vi "Count_looped.vi"(7 "Reset?":bool[](array[boolean]), 11 "Input array":dbl[](array[numeric])) -> (3 "Output array":dbl[](array[numeric]))   [LabVIEW 2018]
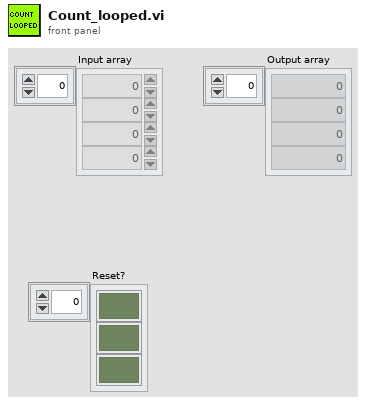
[diagram p1: front panel]
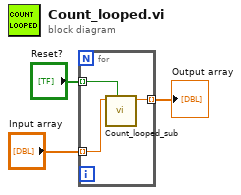
[diagram p0: block diagram]
diagram:
  n1 = for {
    tunnel: "Input array" -> [w5] mode=indexing
    tunnel: "Reset?" -> [w6] mode=indexing
    tunnel: [w4] -> w1 mode=indexing
    n2 = call "Count_looped_sub.vi"("Reset?"=w6, "Input sample"=w5) -> ("Sum of samples"=w4:dbl)  [unwired: 9 in]
  }
  "Output array" <- w1
